vi "Layout Scrollbars.vi"(8 "error in (no error)":errorcluster, 11 "2DArrayManager in":refnum<class "2DArrayManager.lvclass">) -> (0 "error out":errorcluster, 3 "2DArrayManager out":refnum<class "2DArrayManager.lvclass">)   [LabVIEW 2020, in "OOPanel.lvlib" / "2DArrayManager.lvclass"]
uses:
  2DArrayManager.lvclass
  2DArrayManager.lvclass/2DArrayManager.ctl
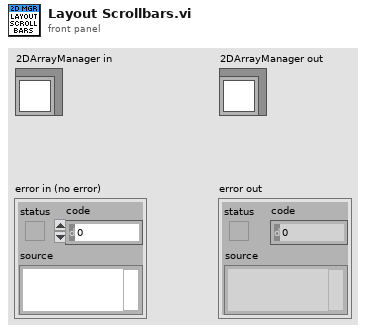
[diagram p1: front panel]
types:
  T1 = typedef "OOPanel.lvlib/2DArrayManager.lvclass/UI Refs.ctl" = cluster{"SubPanels":refnum<vi>[], "Panel VI":refnum<vi>, "Container":refnum<vi>, "H Scroll":refnum<vi>, "V Scroll":refnum<vi>, "Owning VI":refnum<vi>, "FP":refnum<vi>, "Corner":refnum<vi>}
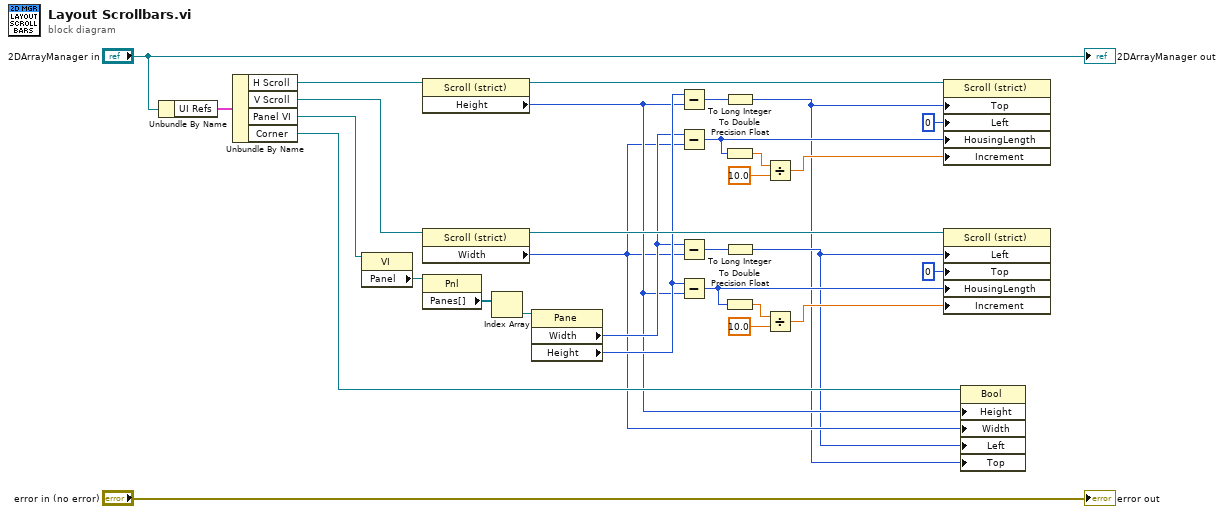
[diagram p0: block diagram]
diagram:
  n1 = Unbundle By Name("2DArrayManager in") -> ("UI Refs"=w8:T1)
  n2 = Unbundle By Name(w8) -> ("H Scroll"=w17:refnum<vi>, "V Scroll"=w28:refnum<vi>, "Panel VI"=w22:refnum<vi>, "Corner"=w5:refnum<vi>)
  n3 = property class="VI"(reference=w22) -> ("Panel"=w29:refnum<vi>)  [unwired: 1 in, 2 out]
  n4 = property class="Scroll (strict)"(reference=w17) -> (reference out=w15:refnum<vi>, "Height"=w4:u32)  [unwired: 1 in, 1 out]
  n5 = property class="Scroll (strict)"(reference=w28) -> (reference out=w27:refnum<vi>, "Width"=w3:u32)  [unwired: 1 in, 1 out]
  n6 = property class="Pnl"(reference=w29) -> ("Panes[]"=w25:refnum<vi>[])  [unwired: 1 in, 2 out]
  n7 = Index Array(array=w25) -> (element=w24:refnum<vi>)  [unwired: 1 in]
  n8 = property class="Pane"(reference=w24) -> ("Width"=w10:u32, "Height"=w16:u32)  [unwired: 1 in, 2 out]
  n9 = Subtract(x=w16, y=w4) -> (x-y=w14:u32)
  n10 = Subtract(x=w10, y=w3) -> (x-y=w7:u32)
  n11 = Subtract(x=w10, y=w3) -> (x-y=w23:u32)
  n12 = Subtract(x=w16, y=w4) -> (x-y=w6:u32)
  n13 = To Long Integer(number=w14) -> (32bit integer=w1:i32)
  n14 = To Double Precision Float(number=w7) -> (double precision float=w11:dbl)
  n15 = To Long Integer(number=w23) -> (32bit integer=w2:i32)
  n16 = To Double Precision Float(number=w6) -> (double precision float=w21:dbl)
  n17 = Divide(x=w11, y=10.0) -> (x/y=w9:dbl)
  n18 = Divide(x=w21, y=10.0) -> (x/y=w19:dbl)
  n19 = property class="Scroll (strict)"(reference=w15, "Top"=w1, "Left"=0 ("Position:Left"), "HousingLength"=w7, "Increment"=w9) -> ()  [unwired: 1 in, 2 out]
  n20 = property class="Scroll (strict)"(reference=w27, "Left"=w2, "Top"=0 ("Position:Top"), "HousingLength"=w6, "Increment"=w19) -> ()  [unwired: 1 in, 2 out]
  n21 = property class="Bool"(reference=w5, "Height"=w4, "Width"=w3, "Left"=w2, "Top"=w1) -> ()  [unwired: 1 in, 2 out]
  "error out" <- "error in (no error)"
  "2DArrayManager out" <- "2DArrayManager in"
